vi "loadOvenData.vi"() -> ()   [LabVIEW 2012]
uses:
  <vilib>/addons/database/Auxilliary.llb/DB Tools Cursor Type.ctl
  <vilib>/addons/database/Connection.llb/DB Tools Open Connec (Path).vi
  <vilib>/addons/database/Connection.llb/Conn Execute.vi
  <vilib>/addons/database/Recordset.llb/Rec Fetch Recordset Data (R).vi
  <vilib>/addons/database/Recordset.llb/Rec Destroy - Connection.vi
  <vilib>/addons/database/Recordset.llb/Rec Fetch Integer Data (R).vi
  <vilib>/addons/database/_DB Variant To Data/Database Variant To Data.xnode
  <vilib>/addons/database/NI_Database_API.lvlib
panel:
  out "Cluster 2":T1
  out "error out 2":errorcluster
  out "data 2":string
  out "AsciiOutput":string
  out "data":string
  in  "Cluster":T1
  out "recordset data":variant[][](array[variant])
  out "error out":errorcluster
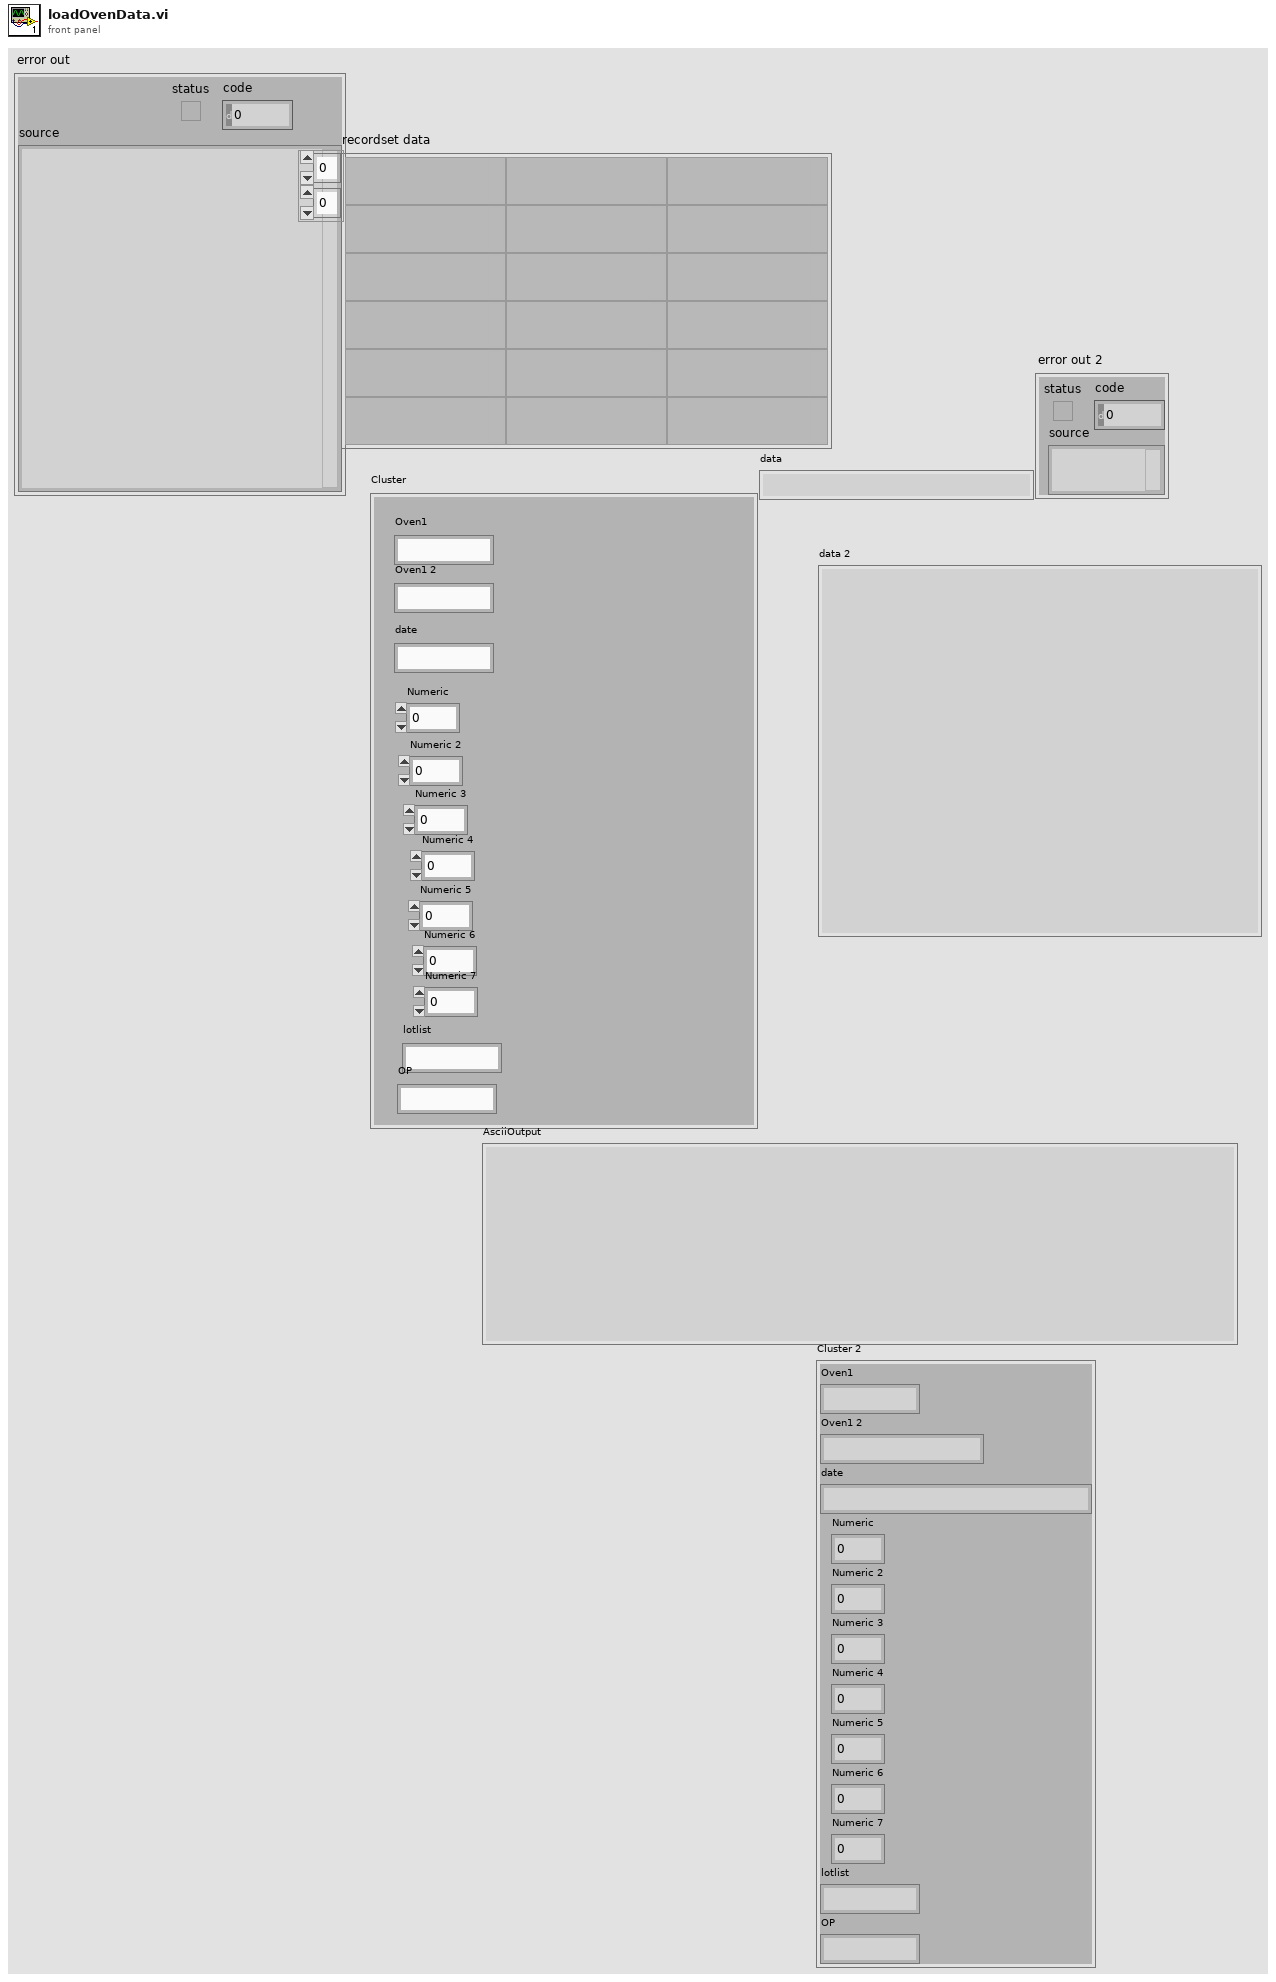
[diagram p1: front panel]
types:
  T1 = cluster{"Oven1":string, "Oven1 2":string, "date":string, "Numeric":dbl, "Numeric 2":dbl, "Numeric 3":dbl, "Numeric 4":dbl, "Numeric 5":dbl, "Numeric 6":dbl, "Numeric 7":dbl, "lotlist":string, "OP":string}
  T2 = typedef "NI_Database_API.lvlib/DB Tools Cursor Type.ctl" = enum16{"forward-only", "keyset", "dynamic", "static"}
  T3 = typedef "NI_Database_API.lvlib/Conn ObjectReference.ctl" = refnum<k1>
  T4 = typedef "NI_Database_API.lvlib/Rec ObjectReference.ctl" = refnum<k1>
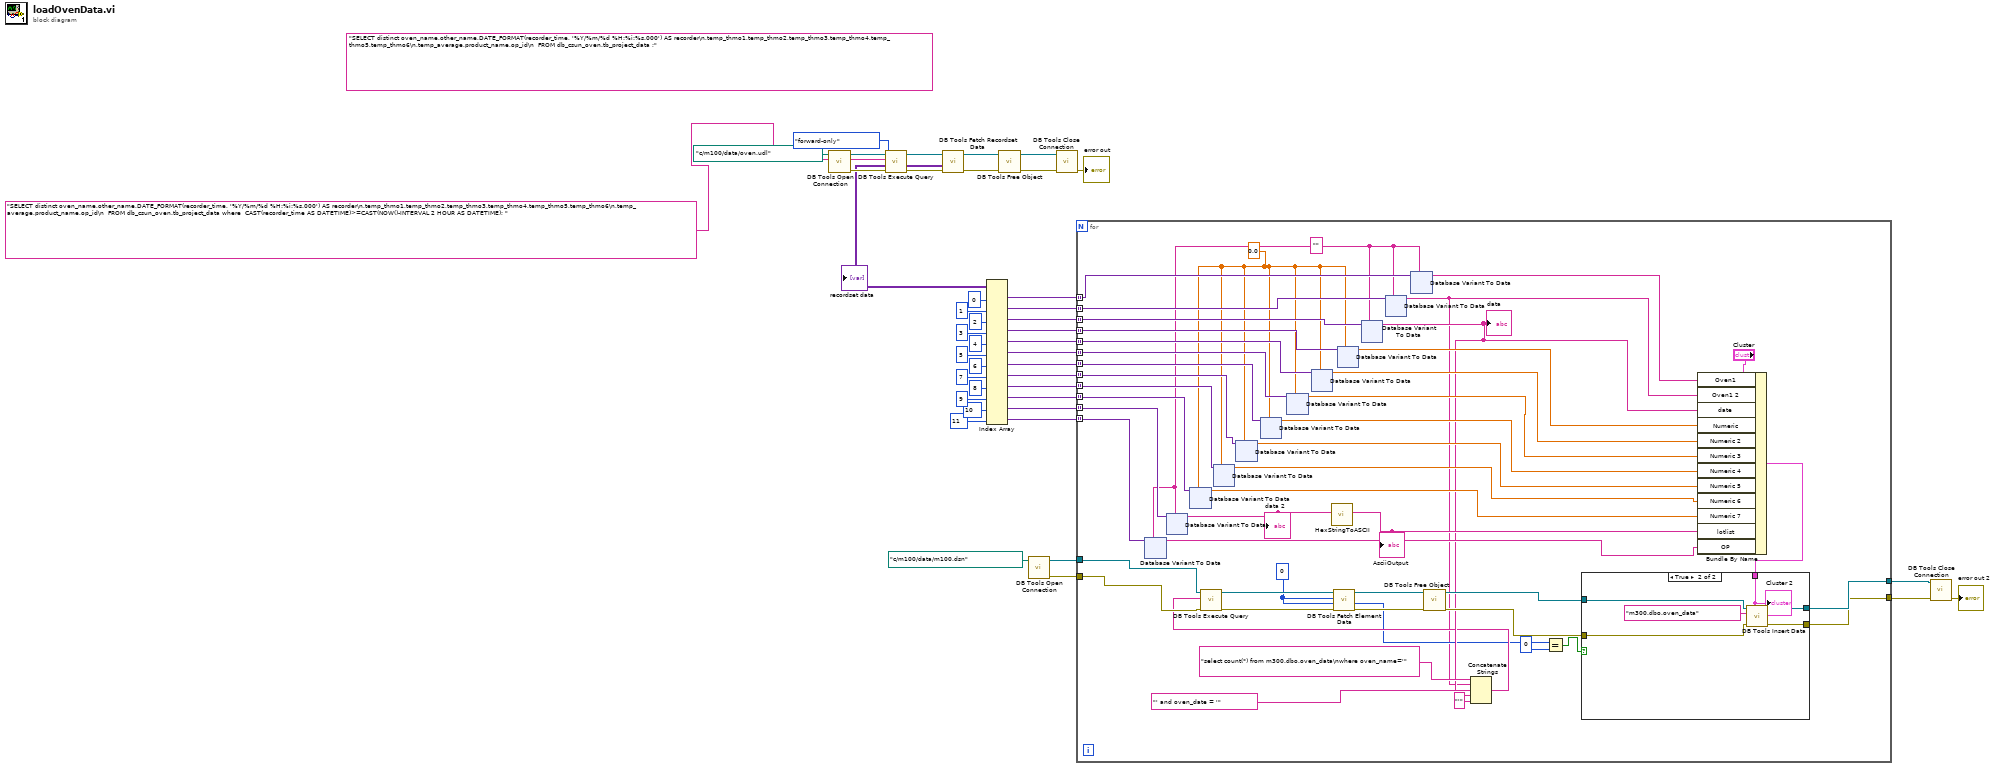
[diagram p0: block diagram]
diagram:
  (unwired) "SELECT distinct oven_name,other_name,DATE_FORMAT(recorder_time, '%Y/%m/%d %H:%i:%s.000') AS recorder\n,temp_thmo1,temp_thmo2,temp_thmo3,temp_thmo4,temp_thmo5,temp_thmo6\n,temp_average,product_name,op_id\n  FROM db_csun_oven.tb_project_data ;" ("SQL query")
  n1 = call-poly <vilib>:"DB Tools Open Connection.vi"("connection information"=path "c:/m100/data/oven.udl") -> ("error out"=w39:errorcluster, "connection reference"=w43:T3)  [unwired: 7 in]
  n2 = call-poly <vilib>:"DB Tools Execute Query.vi"("error in (no error)"=w39, "cursor type"=DB_Tools_Cursor_Type."forward-only", "SQL query"="SELECT distinct oven_name,other_name,DATE_FORMAT(recorder_time, '%Y/%m/%d %H:%i:%s.000') AS recorder\n,temp_thmo1,temp_thmo2,temp_thmo3,temp_thmo4,temp_thmo5,temp_thmo6\n,temp_average,product_name,op_id\n  FROM db_csun_oven.tb_project_data where  CAST(recorder_time AS DATETIME)>=CAST(NOW()-INTERVAL 2 HOUR AS DATETIME); ", "connection reference"=w43) -> ("error out"=w38:errorcluster, "recordset reference"=w42:T4)  [unwired: 4 in]
  n3 = call-poly <vilib>:"DB Tools Fetch Recordset Data.vi"("error in (no error)"=w38, "recordset reference"=w42) -> ("error out"=w37:errorcluster, "recordset data"=w32:variant[][], "recordset reference out"=w41:T4)  [unwired: 3 in]
  "recordset data" <- w32
  n4 = Index Array(array=w32, index (col) #1=0 ("disabled index (col)"), index (col) #2=1 ("index (col)"), index (col) #3=2 ("index (col)"), index (col) #4=3 ("index (col)"), index (col) #5=4 ("index (col)"), index (col) #6=5 ("index (col)"), index (col) #7=6 ("index (col)"), index (col) #8=7 ("index (col)"), index (col) #9=8 ("index (col)"), index (col) #10=9 ("index (col)"), index (col) #11=10 ("index (col)"), index (col) #12=11 ("index (col)")) -> (element #1=w19:variant[], element #2=w18:variant[], element #3=w17:variant[], element #4=w16:variant[], element #5=w15:variant[], element #6=w14:variant[], element #7=w13:variant[], element #8=w12:variant[], element #9=w11:variant[], element #10=w10:variant[], element #11=w9:variant[], element #12=w8:variant[])  [unwired: 12 in]
  n5 = call-poly <vilib>:"DB Tools Free Object.vi"("error in (no error)"=w37, "recordset reference"=w41) -> ("error out"=w36:errorcluster, "connection reference"=w40:T3)  [unwired: 8 in]
  n6 = call-poly <vilib>:"DB Tools Open Connection.vi"("connection information"=path "c:/m100/data/m100.dsn") -> ("error out"=w5:errorcluster, "connection reference"=w6:T3)  [unwired: 7 in]
  n7 = call <vilib>:"DB Tools Close Connection.vi"("error in (no error)"=w36, "connection reference"=w40) -> ("error out"=→"error out":errorcluster)  [unwired: 5 in]
  n8 = for {
    tunnel: w19 -> [w90] mode=indexing
    tunnel: w18 -> [w89] mode=indexing
    tunnel: w17 -> [w88] mode=indexing
    tunnel: w16 -> [w87] mode=indexing
    tunnel: w15 -> [w86] mode=indexing
    tunnel: w14 -> [w85] mode=indexing
    tunnel: w13 -> [w84] mode=indexing
    tunnel: w12 -> [w83] mode=indexing
    tunnel: w11 -> [w82] mode=indexing
    tunnel: w10 -> [w81] mode=indexing
    tunnel: w9 -> [w80] mode=indexing
    tunnel: w8 -> [w79] mode=indexing
    tunnel: w6 -> [w60]
    tunnel: w5 -> [w59]
    tunnel: [w65] -> w4
    tunnel: [w64] -> w3
    w49 = 0
    w78 = 0.0
    w77 = ""
    n9 = xnode "Database Variant To Data"("database variant"=w79, "type"=w77) -> ("data"=w68:string)  [unwired: 1 in, 1 out]
    n10 = xnode "Database Variant To Data"("database variant"=w80, "type"=w77) -> ("data"=w67:string)  [unwired: 1 in, 1 out]
    "data 2" <- w67
    n11 = xnode "Database Variant To Data"("database variant"=w81, "type"=w78) -> ("data"=w69:dbl)  [unwired: 1 in, 1 out]
    n12 = xnode "Database Variant To Data"("database variant"=w82, "type"=w78) -> ("data"=w70:dbl)  [unwired: 1 in, 1 out]
    n13 = xnode "Database Variant To Data"("database variant"=w83, "type"=w78) -> ("data"=w71:dbl)  [unwired: 1 in, 1 out]
    n14 = xnode "Database Variant To Data"("database variant"=w84, "type"=w78) -> ("data"=w72:dbl)  [unwired: 1 in, 1 out]
    n15 = xnode "Database Variant To Data"("database variant"=w85, "type"=w78) -> ("data"=w73:dbl)  [unwired: 1 in, 1 out]
    n16 = xnode "Database Variant To Data"("database variant"=w86, "type"=w78) -> ("data"=w74:dbl)  [unwired: 1 in, 1 out]
    n17 = call "HexStringToASCII.vi"("HexIStringnput"=w67) -> ("AsciiOutput"=w66:string)  [unwired: 10 in]
    "AsciiOutput" <- w66
    n18 = xnode "Database Variant To Data"("database variant"=w87, "type"=w78) -> ("data"=w75:dbl)  [unwired: 1 in, 1 out]
    n19 = xnode "Database Variant To Data"("database variant"=w88, "type"=w77) -> ("data"=w52:string)  [unwired: 1 in, 1 out]
    "data" <- w52
    n20 = xnode "Database Variant To Data"("database variant"=w89, "type"=w77) -> ("data"=w45:string)  [unwired: 1 in, 1 out]
    n21 = xnode "Database Variant To Data"("database variant"=w90, "type"=w77) -> ("data"=w44:string)  [unwired: 1 in, 1 out]
    n22 = Concatenate Strings("select count(*) from m300.dbo.oven_data\nwhere oven_name='", w45, "' and oven_date = '" ("string"), w52, "'" ("string")) -> (w50:string)
    n23 = call-poly <vilib>:"DB Tools Execute Query.vi"("error in (no error)"=w59, "SQL query"=w50, "connection reference"=w60) -> ("error out"=w58:errorcluster, "recordset reference"=w62:T4)  [unwired: 5 in]
    n24 = call-poly <vilib>:"DB Tools Fetch Element Data.vi"("error in (no error)"=w58, "type"=w49, "column index"=w49, "recordset reference"=w62) -> ("error out"=w57:errorcluster, "data"=w48:i32, "recordset reference out"=w61:T4)  [unwired: 3 in]
    n25 = call-poly <vilib>:"DB Tools Free Object.vi"("error in (no error)"=w57, "recordset reference"=w61) -> ("error out"=w55:errorcluster, "connection reference"=w56:T3)  [unwired: 8 in]
    n26 = Equal?(x=w48, y=0) -> (x = y?=w46:bool)
    n27 = Bundle By Name(cluster="Cluster", "Oven1"=w44, "Oven1 2"=w45, "date"=w52, "Numeric"=w75, "Numeric 2"=w74, "Numeric 3"=w73, "Numeric 4"=w72, "Numeric 5"=w71, "Numeric 6"=w70, "Numeric 7"=w69, "lotlist"=w66, "OP"=w68) -> (w63:T1)
    n28 = case shown="True" w46 {
      tunnel: [w92 w98] -> w65
      tunnel: [w91 w97] -> w64
      tunnel: w63 -> [_ w95]
      tunnel: w56 -> [w92 w94]
      tunnel: w55 -> [w91 w93]
      frame False {
      }
      frame True {
        n29 = call <vilib>:"DB Tools Insert Data.vi"("data"=w95, "error in (no error)"=w93, "table"="m300.dbo.oven_data", "connection reference"=w94) -> ("error out"=w97:errorcluster, "connection reference out"=w98:T3)  [unwired: 6 in]
        "Cluster 2" <- w95
      }
    }
  }
  n30 = call <vilib>:"DB Tools Close Connection.vi"("error in (no error)"=w3, "connection reference"=w4) -> ("error out"=→"error out 2":errorcluster)  [unwired: 5 in]
